vi "FGV LabBase Index.vi"(6 "Aktion":T1, 8 "error in (no error)":errorcluster caption="Fehler (Eingang, kein Fehler)", 11 "Index Nr. Start:":u32 caption="SPEC#:") -> (0 "error out":errorcluster caption="Fehler (Ausgang)", 3 "Index Nr. Start:":u32)   [LabVIEW 2020, in "LogKonfig.lvlib"]
uses:
  Aktion LabBaseIndex.ctl
  LogKonfig.lvlib
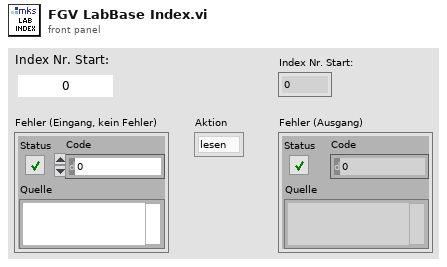
[diagram p1: front panel]
types:
  T1 = typedef "LogKonfig.lvlib/Aktion LabBaseIndex.ctl" = enum16{"lesen", "schreiben"}
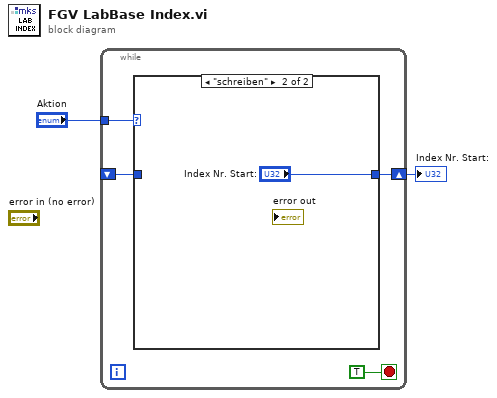
[diagram p0: block diagram]
diagram:
  n1 = while {
    tunnel: "Aktion" -> [w5]
    shift-right: [w4] -> w1
    shift-left: _ -> [w3]
    stop <- TRUE stop-if-true
    n2 = case shown="\"schreiben\"" w5 {
      tunnel: [w7 "Index Nr. Start:"] -> w4
      tunnel: w3 -> [w7 _]
      frame "lesen" {
      }
      frame "schreiben" {
      }
    }
  }
  "Index Nr. Start:" <- w1
